vi "Initialise Checkbox.vi"(8 "error in (no error)":errorcluster, 10 "Check Value (F)":bool, 11 "MCListbox with Checkboxes in":refnum<class "MCListbox with Checkboxes.lvclass">) -> (0 "error out":errorcluster, 3 "MCListbox with Checkboxes out":refnum<class "MCListbox with Checkboxes.lvclass">)   [LabVIEW 2016, in "MCListbox with Checkboxes.lvclass"]
uses:
  MCListbox with Checkboxes.lvclass
  MCListbox with Checkboxes.lvclass/MCListbox with Checkboxes.ctl
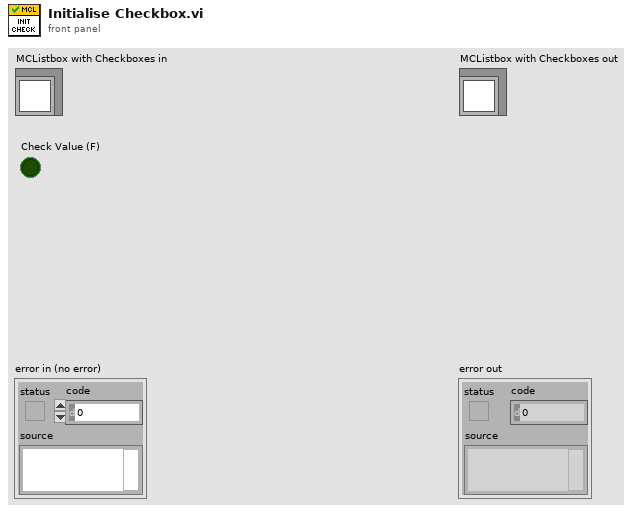
[diagram p1: front panel]
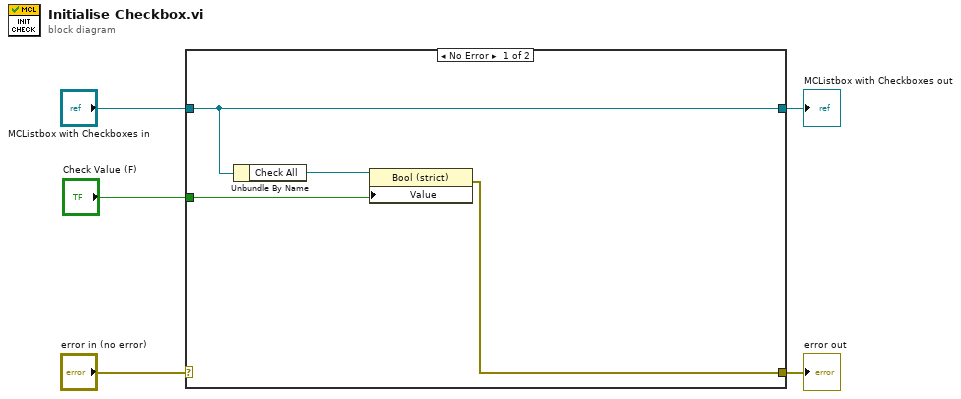
[diagram p0: block diagram]
diagram:
  n1 = case shown="No Error" "error in (no error)" {
    selector: "error in (no error)" -> [_ w11]
    tunnel: [w6 w11] -> w4
    tunnel: [w9 w10] -> w2
    tunnel: "MCListbox with Checkboxes in" -> [w9 w10]
    tunnel: "Check Value (F)" -> [w7 _]
    frame No Error {
      n2 = Unbundle By Name(w9) -> ("Check All"=w8:refnum<vi>)
      n3 = property class="Bool (strict)"(reference=w8, "Value"=w7) -> (error out=w6:errorcluster)  [unwired: 1 in, 1 out]
    }
    frame Error {
    }
  }
  "error out" <- w4
  "MCListbox with Checkboxes out" <- w2
